vi "connect PG server.vi"(8 "error in (no error)":errorcluster, 11 "SP in":refnum<class "Save messages PGserver.lvclass">) -> (0 "error out":errorcluster, 2 "conn_out":u64, 3 "SP out":refnum<class "Save messages PGserver.lvclass">)   [LabVIEW 2019, in "Save messages PGserver.lvclass"]
uses:
  Save messages PGserver.lvclass
  Save messages PGserver.lvclass/Save messages PGserver.ctl
  PostgreSQL2LabVIEW/libpqlv/src/PQfinish.vi
  PostgreSQL2LabVIEW/libpqlv/src/PQconnectdb.vi
  PostgreSQL2LabVIEW/libpqlv/src/PQerrorMessage.vi
  PostgreSQL2LabVIEW/libpqlv/src/PQstatus.vi
  <vilib>/dlg_ctls.llb/Space Constant.vi
  PostgreSQL2LabVIEW/libpqUtility64/libpqutility64.lvlib
  PostgreSQL2LabVIEW/libpqUtility/libpqutility.lvlib
panel:
  out "PQStatus":T1(ring)
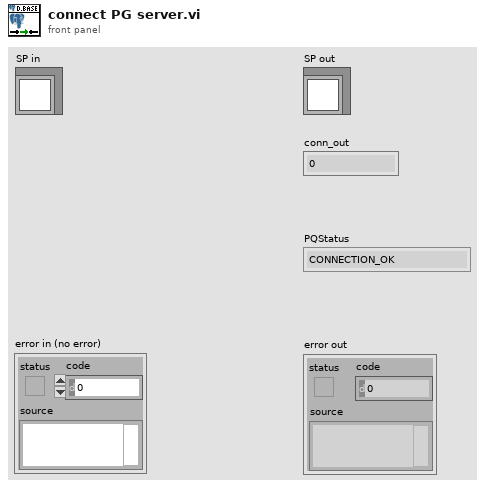
[diagram p1: front panel]
types:
  T1 = enum32{"CONNECTION_OK", "CONNECTION_BAD", "CONNECTION_STARTED", "CONNECTION_MADE", "CONNECTION_AWAITING_RESPONSE", "CONNECTION_AUTH_OK", "CONNECTION_SETENV", "CONNECTION_SSL_STARTUP", "CONNECTION_NEEDED"}
  T2 = typedef "PostgreSQL.lvlib/Coninfo.ctl" = cluster{"host":string, "port":string, "client_encoding":string, "dbname":string, "user":string, "password":string}
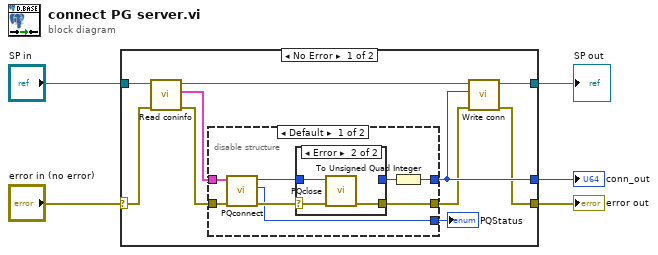
[diagram p0: block diagram]
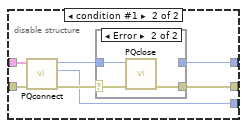
[diagram p3: hidden frame]
diagram:
  n1 = case shown="No Error" "error in (no error)" {
    selector: "error in (no error)" -> [w13 w41]
    tunnel: [w9 w41] -> w4
    tunnel: [w12 w42] -> w2
    tunnel: "SP in" -> [w15 w42]
    tunnel: [w11 _] -> w1
    frame No Error {
      n2 = call "Read coninfo.vi"("error in (no error)"=w13, "SP in"=w15) -> ("error out"=w8:errorcluster, "conninfo"=w14:T2, "SP out"=w7:refnum<class "Save messages PGserver.lvclass">)  [unwired: 7 in]
      n3 = disable-structure shown="Default" {
        disable-tunnel: w14 -> [w23 w35]
        disable-tunnel: [w17 w34] -> w11
        disable-tunnel: [w21 w33] -> w10
        disable-tunnel: w8 -> [w20 w32]
        disable-tunnel: [w16 w29] -> w6
        frame condition #0 (active) {
          n4 = call "PQconnect.vi"("error in (no error)"=w20, "conninfo"=w23) -> ("error out"=w18:errorcluster, "PQStatus"=w16:T1, "conn"=w19:u32)  [unwired: 7 in]
          n5 = case shown="Error" w18 {
            selector: w18 -> [w24 w27]
            tunnel: w19 -> [w25 w28]
            tunnel: [w25 _] -> w22
            tunnel: [w24 w26] -> w21
            frame No Error {
            }
            frame Error {
              n6 = call "PQclose.vi"("error in (no error)"=w27, "conn"=w28) -> ("error out"=w26:errorcluster)  [unwired: 9 in]
            }
          }
          n7 = To Unsigned Quad Integer(1:w22) -> (0:w17:u64)
        }
        frame condition #1 {
          n8 = call "PQconnect.vi"("error in (no error)"=w32, "conninfo"=w35) -> ("error out"=w30:errorcluster, "PQStatus"=w29:T1, "conn"=w31:u64)  [unwired: 7 in]
          n9 = case shown="Error" w30 {
            selector: w30 -> [w36 w39]
            tunnel: w31 -> [w37 w40]
            tunnel: [w37 _] -> w34
            tunnel: [w36 w38] -> w33
            frame No Error {
            }
            frame Error {
              n10 = call "PQclose.vi"("error in (no error)"=w39, "conn"=w40) -> ("error out"=w38:errorcluster)  [unwired: 9 in]
            }
          }
        }
      }
      "PQStatus" <- w6
      n11 = call "Write conn.vi"("error in (no error)"=w10, "conn"=w11, "SP in"=w7) -> ("error out"=w9:errorcluster, "SP out"=w12:refnum<class "Save messages PGserver.lvclass">)  [unwired: 7 in]
    }
    frame Error {
    }
  }
  "error out" <- w4
  "SP out" <- w2
  "conn_out" <- w1
